vi "NIIE_Process Template Graphics.vi"(8 "Error":errorcluster, 10 "Match Data":T9, 11 "Data":T1={"Class"={"Ants"=refnum, "Layer"=refnum, "Templates"=refnum, "Icon"=refnum, "Glyph"=refnum, "Settings"=refnum, "Tools"=refnum}, "Ref"={"Add Layer"=refnum, "Remove Layer"=refnum, "Line Text"=[], "Body Text Spec"=refnum, "DNL_Font"=refnum, "glyph path str"=refnum, "templates path str"=refnum, "Arrow Up"=refnum, "Arrow Down"=refnum, "IE VI Ref"=refnum, "Glyphs tree"=refnum, "Templates tree"=refnum, "Layer Icon Text"=refnum, "Layer Template"=refnum, "Clipboard"=refnum, "BW icon in"=refnum, "Color icon in"=refnum, "Layer Clust"=refnum, "Body Text"=refnum, "DNL_Framework Templates"=refnum, "Search Templates"=refnum, "TextMarker"=refnum, "Tab Control"=refnum, "Search Glyphs"=refnum, "Line Color"=refnum, "DNL_Glyphs []"=refnum, "Fill Color"=refnum, "Tools"=refnum, "Glyphs tree"=refnum, "Icon"=refnum, "Preview"=refnum, "Ants"=refnum, "Terminals"=refnum, "menu reference"=refnum, "LayerNames"=[], "GlyphLoadAnimation"=refnum, "TemplateLoadAnimation"=refnum, "refreshGlyphs"=refnum, "refreshTemplates"=refnum}, "Support"={"AntsRect"={"left"=0, "top"=0, "right"=0, "bottom"=0}, "Mouse Move Coords"={"Horizontal"=0, "Vertical"=0}, "Mouse Down Coords"={"Horizontal"=0, "Vertical"=0}, "Temp Coord"={"Horizontal"=0, "Vertical"=0}, "Action"=enum."Default", "Edge Color"=4914962, "Fill Color"=16860, "Mouse Down?"=FALSE, "Draft Mode?"=FALSE, "Temp Icon"=bytes[3102], "CTRL Pressed"=FALSE, "Move Selection?"=FALSE, "AntsRect Orig"={"left"=0, "top"=0, "right"=0, "bottom"=0}, "Text"="", "TM Set?"=FALSE, "Mouse inside icon?"=FALSE, "Tool (old value)"=0, "Pencil Move Color"=0, "Swap Colors?"=FALSE, "Shift pressed?"=FALSE}}) -> (0 "Error Out":errorcluster, 3 "Data Out":T1={"Class"={"Ants"=refnum, "Layer"=refnum, "Templates"=refnum, "Icon"=refnum, "Glyph"=refnum, "Settings"=refnum, "Tools"=refnum}, "Ref"={"Add Layer"=refnum, "Remove Layer"=refnum, "Line Text"=[], "Body Text Spec"=refnum, "DNL_Font"=refnum, "glyph path str"=refnum, "templates path str"=refnum, "Arrow Up"=refnum, "Arrow Down"=refnum, "IE VI Ref"=refnum, "Glyphs tree"=refnum, "Templates tree"=refnum, "Layer Icon Text"=refnum, "Layer Template"=refnum, "Clipboard"=refnum, "BW icon in"=refnum, "Color icon in"=refnum, "Layer Clust"=refnum, "Body Text"=refnum, "DNL_Framework Templates"=refnum, "Search Templates"=refnum, "TextMarker"=refnum, "Tab Control"=refnum, "Search Glyphs"=refnum, "Line Color"=refnum, "DNL_Glyphs []"=refnum, "Fill Color"=refnum, "Tools"=refnum, "Glyphs tree"=refnum, "Icon"=refnum, "Preview"=refnum, "Ants"=refnum, "Terminals"=refnum, "menu reference"=refnum, "LayerNames"=[], "GlyphLoadAnimation"=refnum, "TemplateLoadAnimation"=refnum, "refreshGlyphs"=refnum, "refreshTemplates"=refnum}, "Support"={"AntsRect"={"left"=0, "top"=0, "right"=0, "bottom"=0}, "Mouse Move Coords"={"Horizontal"=0, "Vertical"=0}, "Mouse Down Coords"={"Horizontal"=0, "Vertical"=0}, "Temp Coord"={"Horizontal"=0, "Vertical"=0}, "Action"=enum."Default", "Edge Color"=4914962, "Fill Color"=16860, "Mouse Down?"=FALSE, "Draft Mode?"=FALSE, "Temp Icon"=bytes[3102], "CTRL Pressed"=FALSE, "Move Selection?"=FALSE, "AntsRect Orig"={"left"=0, "top"=0, "right"=0, "bottom"=0}, "Text"="", "TM Set?"=FALSE, "Mouse inside icon?"=FALSE, "Tool (old value)"=0, "Pencil Move Color"=0, "Swap Colors?"=FALSE, "Shift pressed?"=FALSE}})   [LabVIEW 2021]
uses:
  MB CORE/TypeDefs/Cluster_Path&Icon.ctl
  Controls/IE Data.ctl
  Ants/Ants.lvclass
  FakedArray.lvclass
  vi.lib/LabVIEW Icon API/lv_icon/Classes/Icon/Icon.lvclass
  Icon Library/Glyph.lvclass
  Settings/Settings.lvclass
  Tools/Tools Paint.lvclass
  Controls/IE Classes.ctl
  Controls/References Cluster.ctl
  Controls/SupportClass.ctl
  <vilib>/Utility/miscctls.llb/LVPoint32TypeDef.ctl
  Controls/ENUM_SupportClass_Action.ctl
  vi.lib/LabVIEW Icon API/lv_icon/Controls/IEColor.ctl
  vi.lib/LabVIEW Icon API/lv_icon/Controls/Pathes.ctl
  Global Variables/NIIE_Global Data.vi
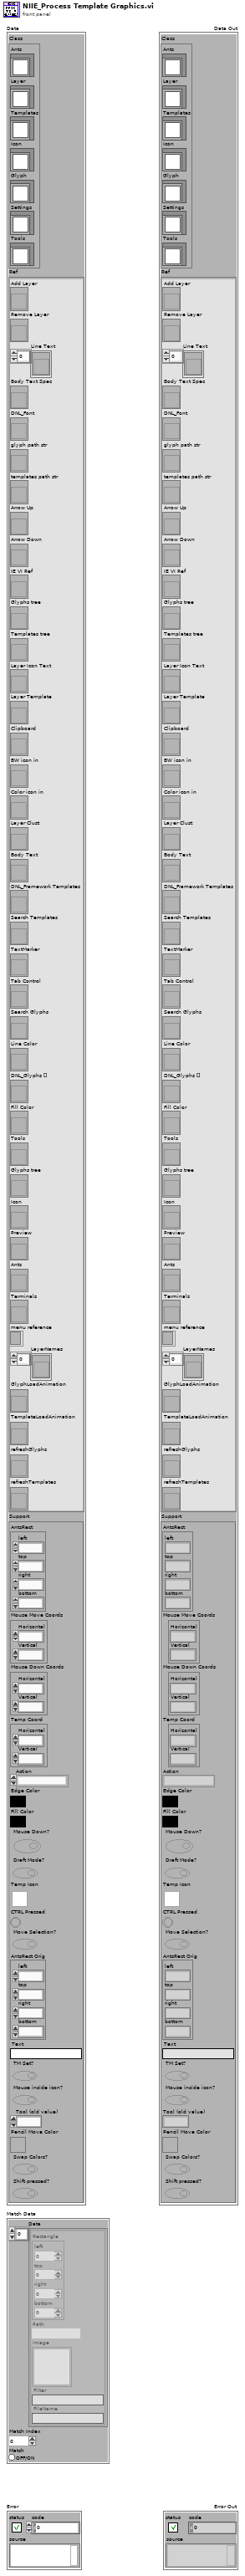
[diagram p1: front panel]
types:
  T1 = typedef "IE Data.ctl" = cluster{"Class":T2, "Ref":T3, "Support":T4}
  T2 = typedef "IE Classes.ctl" = cluster{"Ants":refnum<class "Ants.lvclass">, "Layer":refnum<class "FakedArray.lvclass">, "Templates":refnum<class "FakedArray.lvclass">, "Icon":refnum<class "Icon.lvclass">, "Glyph":refnum<class "Glyph.lvclass">, "Settings":refnum<class "Settings.lvclass">, "Tools":refnum<class "Tools Paint.lvclass">}
  T3 = typedef "References Cluster.ctl" = cluster{"Add Layer":refnum<vi>, "Remove Layer":refnum<vi>, "Line Text":refnum<vi>[], "Body Text Spec":refnum<vi>, "DNL_Font":refnum<vi>, "glyph path str":refnum<vi>, "templates path str":refnum<vi>, "Arrow Up":refnum<vi>, "Arrow Down":refnum<vi>, "IE VI Ref":refnum<vi>, "Glyphs tree":refnum<vi>, "Templates tree":refnum<vi>, "Layer Icon Text":refnum<vi>, "Layer Template":refnum<vi>, "Clipboard":refnum<vi>, "BW icon in":refnum<vi>, "Color icon in":refnum<vi>, "Layer Clust":refnum<vi>, "Body Text":refnum<vi>, "DNL_Framework Templates":refnum<vi>, "Search Templates":refnum<vi>, "TextMarker":refnum<vi>, "Tab Control":refnum<vi>, "Search Glyphs":refnum<vi>, "Line Color":refnum<vi>, "DNL_Glyphs []":refnum<vi>, "Fill Color":refnum<vi>, "Tools":refnum<vi>, "Glyphs tree":refnum<vi>, "Icon":refnum<vi>, "Preview":refnum<vi>, "Ants":refnum<vi>, "Terminals":refnum<vi>, "menu reference":refnum<k9>, "LayerNames":refnum<vi>[], "GlyphLoadAnimation":refnum<vi>, "TemplateLoadAnimation":refnum<vi>, "refreshGlyphs":refnum<vi>, "refreshTemplates":refnum<vi>}
  T4 = typedef "SupportClass.ctl" = cluster{"AntsRect":cluster{"left":i16, "top":i16, "right":i16, "bottom":i16}, "Mouse Move Coords":T5, "Mouse Down Coords":T5, "Temp Coord":T5, "Action":T6, "Edge Color":T7, "Fill Color":T7, "Mouse Down?":bool, "Draft Mode?":bool, "Temp Icon":picture, "CTRL Pressed":bool, "Move Selection?":bool, "AntsRect Orig":cluster{"left":i16, "top":i16, "right":i16, "bottom":i16}, "Text":string, "TM Set?":bool, "Mouse inside icon?":bool, "Tool (old value)":u32, "Pencil Move Color":u32, "Swap Colors?":bool, "Shift pressed?":bool}
  T5 = typedef "LVPoint32TypeDef.ctl" = cluster{"Horizontal":i32, "Vertical":i32}
  T6 = typedef "ENUM_SupportClass_Action.ctl" = enum16{"Default", "Move Selection", "Glyph Library", "Tool"}
  T7 = typedef "IEColor.ctl" = u32
  T8 = typedef "Cluster_Path&Icon.ctl" = cluster{"Rectangle":cluster{"left":i16, "top":i16, "right":i16, "bottom":i16}, "Path":path, "Image":picture, "Filter":string, "FileName":string}
  T9 = cluster{"Data":T8[], "Match Index":i32, "Match":bool}
  T10 = typedef "Pathes.ctl" = enum16{"Root Path", "Icon Templates", "Icon Templates VI", "Icon Templates Lib", "Glyphs"}
  T11 = cluster{"LayerIcon":picture, "LayerName":string, "Opacity":u8, "Visibility?":bool}
  T12 = typedef "Cluster_Layer Data.ctl" = cluster{"LayerIcon":picture, "LayerName":string, "Opacity":u8, "Visibility?":bool}
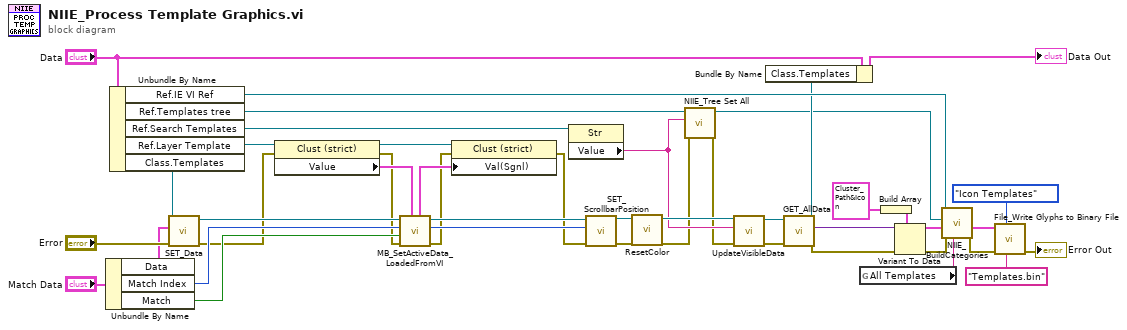
[diagram p0: block diagram]
diagram:
  n1 = Unbundle By Name("Match Data") -> ("Data"=w14:T8[], "Match Index"=w41:i32, "Match"=w40:bool)
  n2 = Unbundle By Name("Data") -> ("Ref.IE VI Ref"=w28:refnum<vi>, "Ref.Templates tree"=w4:refnum<vi>, "Ref.Search Templates"=w15:refnum<vi>, "Ref.Layer Template"=w12:refnum<vi>, "Class.Templates"=w32:refnum<class "FakedArray.lvclass">)
  n3 = call-dynamic "SET_Data.vi"("Error"="Error", "Data"=w14, "FakedArray"=w32) -> ("Error Out"=w7:errorcluster, "FakedArray Out"=w43:refnum<class "FakedArray.lvclass">)  [unwired: 7 out]
  n4 = property class="Clust (strict)"(reference=w12, error in=w7) -> (reference out=w13:refnum<vi>, error out=w6:errorcluster, "Value"=w11:T11)
  n5 = call "MB_SetActiveData_LoadedFromVI.vi"("Layer Data"=w11, "Error"=w6, "Match?"=w40, "Match Index"=w41, "FakedArray"=w43) -> ("Error Out"=w8:errorcluster, "Position Scrollbar Out"=w37:i32, "FakedArray Out"=w38:refnum<class "FakedArray.lvclass">, "Layer Data Out"=w10:T12)  [unwired: 3 out]
  n6 = property class="Clust (strict)"(reference=w13, error in=w8, "Val(Sgnl)"=w10) -> (error out=w9:errorcluster)  [unwired: 1 out]
  n7 = property class="Str"(reference=w15) -> ("Value"=w5:string)  [unwired: 1 in, 2 out]
  n8 = call-dynamic "SET_ScrollbarPosition.vi"("error in (no error)"=w9, "Scrollbar Position"=w37, "FakedArray.lvclass in"=w38) -> ("error out"=w35:errorcluster, "FakedArray.lvclass out"=w34:refnum<class "FakedArray.lvclass">)  [unwired: 7 out]
  n9 = call "ResetColor.vi"("error in (no error)"=w35, "FakedArray in"=w34) -> ("error out"=w2:errorcluster, "FakedArray out"=w33:refnum<class "FakedArray.lvclass">)  [unwired: 8 out]
  n10 = call "NIIE_Tree Set All.vi"("Error"=w2, "Value"=w5, "TreeControl"=w4) -> ("Error Out"=w1:errorcluster, "TreeControl Out"=w3:refnum<vi>)  [unwired: 7 in]
  n11 = call-dynamic "UpdateVisibleData.vi"("Error"=w1, "Keyword"=w5, "FakedArray"=w33) -> ("Error Out"=w26:errorcluster, "FakedArray Out"=w27:refnum<class "FakedArray.lvclass">)  [unwired: 2 in, 5 out]
  n12 = call-dynamic "GET_AllData.vi"("error in (no error)"=w26, "FakedArray.lvclass in"=w27) -> ("error out"=w20:errorcluster, "Data"=w22:variant, "FakedArray.lvclass out"=w25:refnum<class "FakedArray.lvclass">)  [unwired: 7 out]
  n13 = Bundle By Name(cluster="Data", "Class.Templates"=w25) -> (→"Data Out":T1)
  n14 = global read "NIIE_Global Data.vi" "All Templates"() -> (w36:string)
  n15 = Build Array(T8 {"Rectangle"={"left"=0, "top"=0, "right"=0, "bottom"=0}, "Path"=path "", "Image"=bytes[0], "Filter"="", "FileName"=""}) -> (w23:T8[])
  n16 = Variant To Data(error in=w20, type=w23, Variant=w22) -> (data=w21:T8[], error out=w19:errorcluster)
  n17 = call "NIIE_BuildCategories.vi"("Main Item"=w36, "Error"=w19, "IconTemplates"=w21, "Tree"=w3, "VI IE Ref"=w28) -> ("Error Out"=w16:errorcluster, "IconTemplates Out"=w18:T8[])  [unwired: 5 out]
  n18 = call "File_Write Glyphs to Binary File.vi"("File Name"="Templates.bin", "Path"=Pathes."Icon Templates", "Error"=w16, "Graphics []"=w18) -> ("Error Out"=→"Error Out":errorcluster)  [unwired: 7 out]
